vi "Create.vi"(8 "error in (no error)":errorcluster) -> (0 "error out":errorcluster, 3 "Dashed Filter":refnum<class "Dashed Filter.lvclass">)   [LabVIEW 2020, in "Dashed Filter.lvclass"]
uses:
  Dashed Filter.lvclass
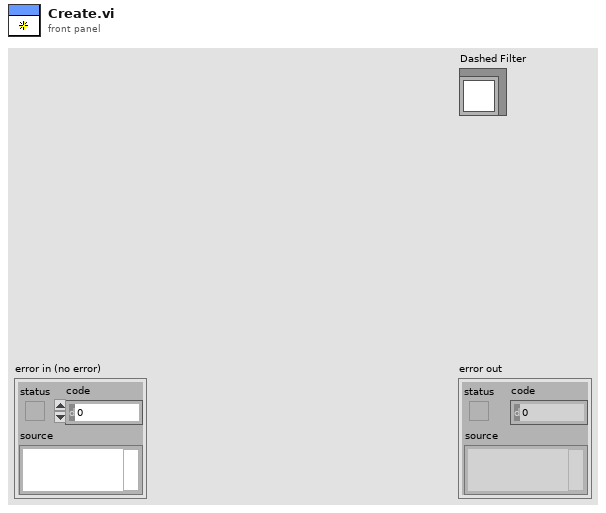
[diagram p1: front panel]
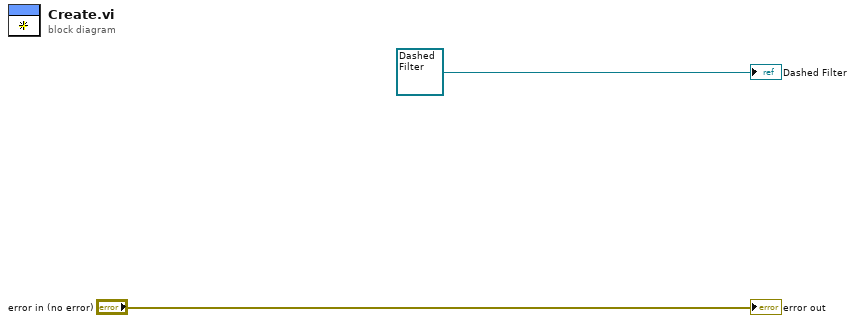
[diagram p0: block diagram]
diagram:
  "error out" <- "error in (no error)"
  "Dashed Filter" <- refnum<class "Dashed Filter.lvclass"> refnum ("Dashed Filter")
